vi "5.1-Forebrain Functional Global for Act neuron.vi"(1 "4.1- Midbrain Act Data":T1, 2 "Command":T3(ring)) -> (0 "6.1.8-Forebrain Act Neuron Data":T2)   [LabVIEW 2010]
uses:
  6-OCU Neurons/6.1.11- Forbrain and midbrain Act neuron.ctl
  4-High Neurons/4.1-Midbrain Act Data.ctl
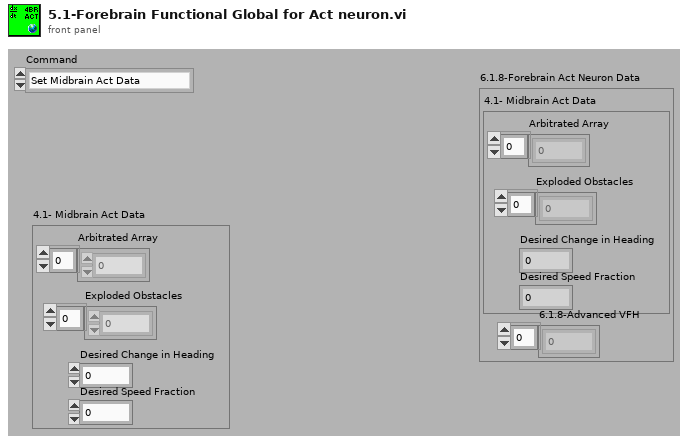
[diagram p1: front panel]
types:
  T1 = typedef "4.1-Midbrain Act Data.ctl" = cluster{"Arbitrated Array":sgl[], "Exploded Obstacles":sgl[], "Desired Change in Heading":sgl, "Desired Speed Fraction":sgl}
  T2 = typedef "6.1.11- Forbrain and midbrain Act neuron.ctl" = cluster{"4.1- Midbrain Act Data":T1, "6.1.8-Advanced VFH":dbl[]}
  T3 = enum16{"Set Midbrain Act Data", "Set Forebrain Act Data", "Read Act Data"}
  T4 = typedef "4.1.2-Act Neuron TD.ctl" = cluster{"Speed By Path":sgl[]}
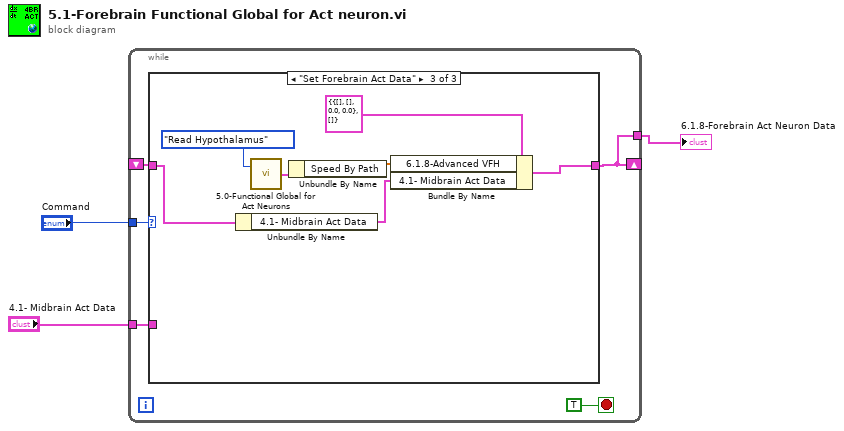
[diagram p0: block diagram]
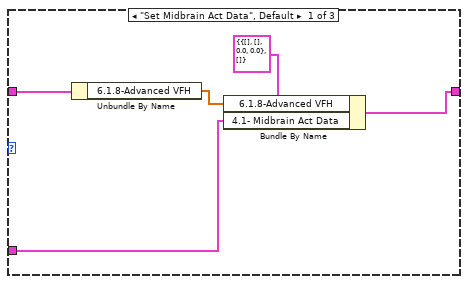
[diagram p2: hidden frame]
diagram:
  n1 = while {
    tunnel: "Command" -> [w7]
    shift-right: [w4] -> _
    shift-left: _ -> [w6]
    tunnel: "4.1- Midbrain Act Data" -> [w5]
    tunnel: [w4] -> w1
    stop <- TRUE stop-if-true
    n2 = case shown="\"Set Forebrain Act Data\"" w7 {
      tunnel: [w9 w14 w17] -> w4
      tunnel: w6 -> [w13 w14 w16]
      tunnel: w5 -> [w10 _ _]
      frame "Set Midbrain Act Data", Default {
        n3 = Unbundle By Name(w13) -> ("6.1.8-Advanced VFH"=w11:dbl[])
        n4 = Bundle By Name(cluster=T2 {"4.1- Midbrain Act Data"={"Arbitrated Array"=[], "Exploded Obstacles"=[], "Desired Change in Heading"=0.0, "Desired Speed Fraction"=0.0}, "6.1.8-Advanced VFH"=[]} ("6.1.8-Forebrain Act Neuron Data"), "6.1.8-Advanced VFH"=w11, "4.1- Midbrain Act Data"=w10) -> (w9:T2)
      }
      frame "Read Act Data" {
      }
      frame "Set Forebrain Act Data" {
        n5 = Unbundle By Name(w16) -> ("4.1- Midbrain Act Data"=w15:T1)
        n6 = call "5.0-Functional Global for Act Neurons.vi"("Mode"=enum16{"Set Hypothalamus", "Read Hypothalamus"}."Read Hypothalamus") -> ("Output Act Neurons"=w19:T4)  [unwired: 1 in]
        n7 = Unbundle By Name(w19) -> ("Speed By Path"=w18:sgl[])
        n8 = Bundle By Name(cluster=T2 {"4.1- Midbrain Act Data"={"Arbitrated Array"=[], "Exploded Obstacles"=[], "Desired Change in Heading"=0.0, "Desired Speed Fraction"=0.0}, "6.1.8-Advanced VFH"=[]} ("6.1.8-Forebrain Act Neuron Data"), "6.1.8-Advanced VFH"=w18, "4.1- Midbrain Act Data"=w15) -> (w17:T2)
      }
    }
  }
  "6.1.8-Forebrain Act Neuron Data" <- w1
